vi "Make DriveBase Curves.vi"() -> ()   [LabVIEW 2020]
uses:
  Motor Type.ctl
panel:
  in  "Count":dbl
  in  "Robot Characterization":T1={"Total Mass"=68.0388555, "Wheel Friction"=1.0, "Wheel Diameter"=0.15239999999999998}
  out "Accel vs Distance for T seconds":T2(graph)
  out "Speed vs Distance for T seconds":T3(graph)
  in  "Ratio":dbl
  in  "Masses":T4(array[cluster])
  out "Accel vs Distance for T seconds":T2(graph)
  in  "Loop Time":dbl[unit]=1.0
  out "Speed vs Distance for T seconds":T3(graph)
  in  "Ratios":dbl[](array[numeric])
  in  "Motor Type":T5=enum."Neo"
  # "Robot Sprint for this many seconds"
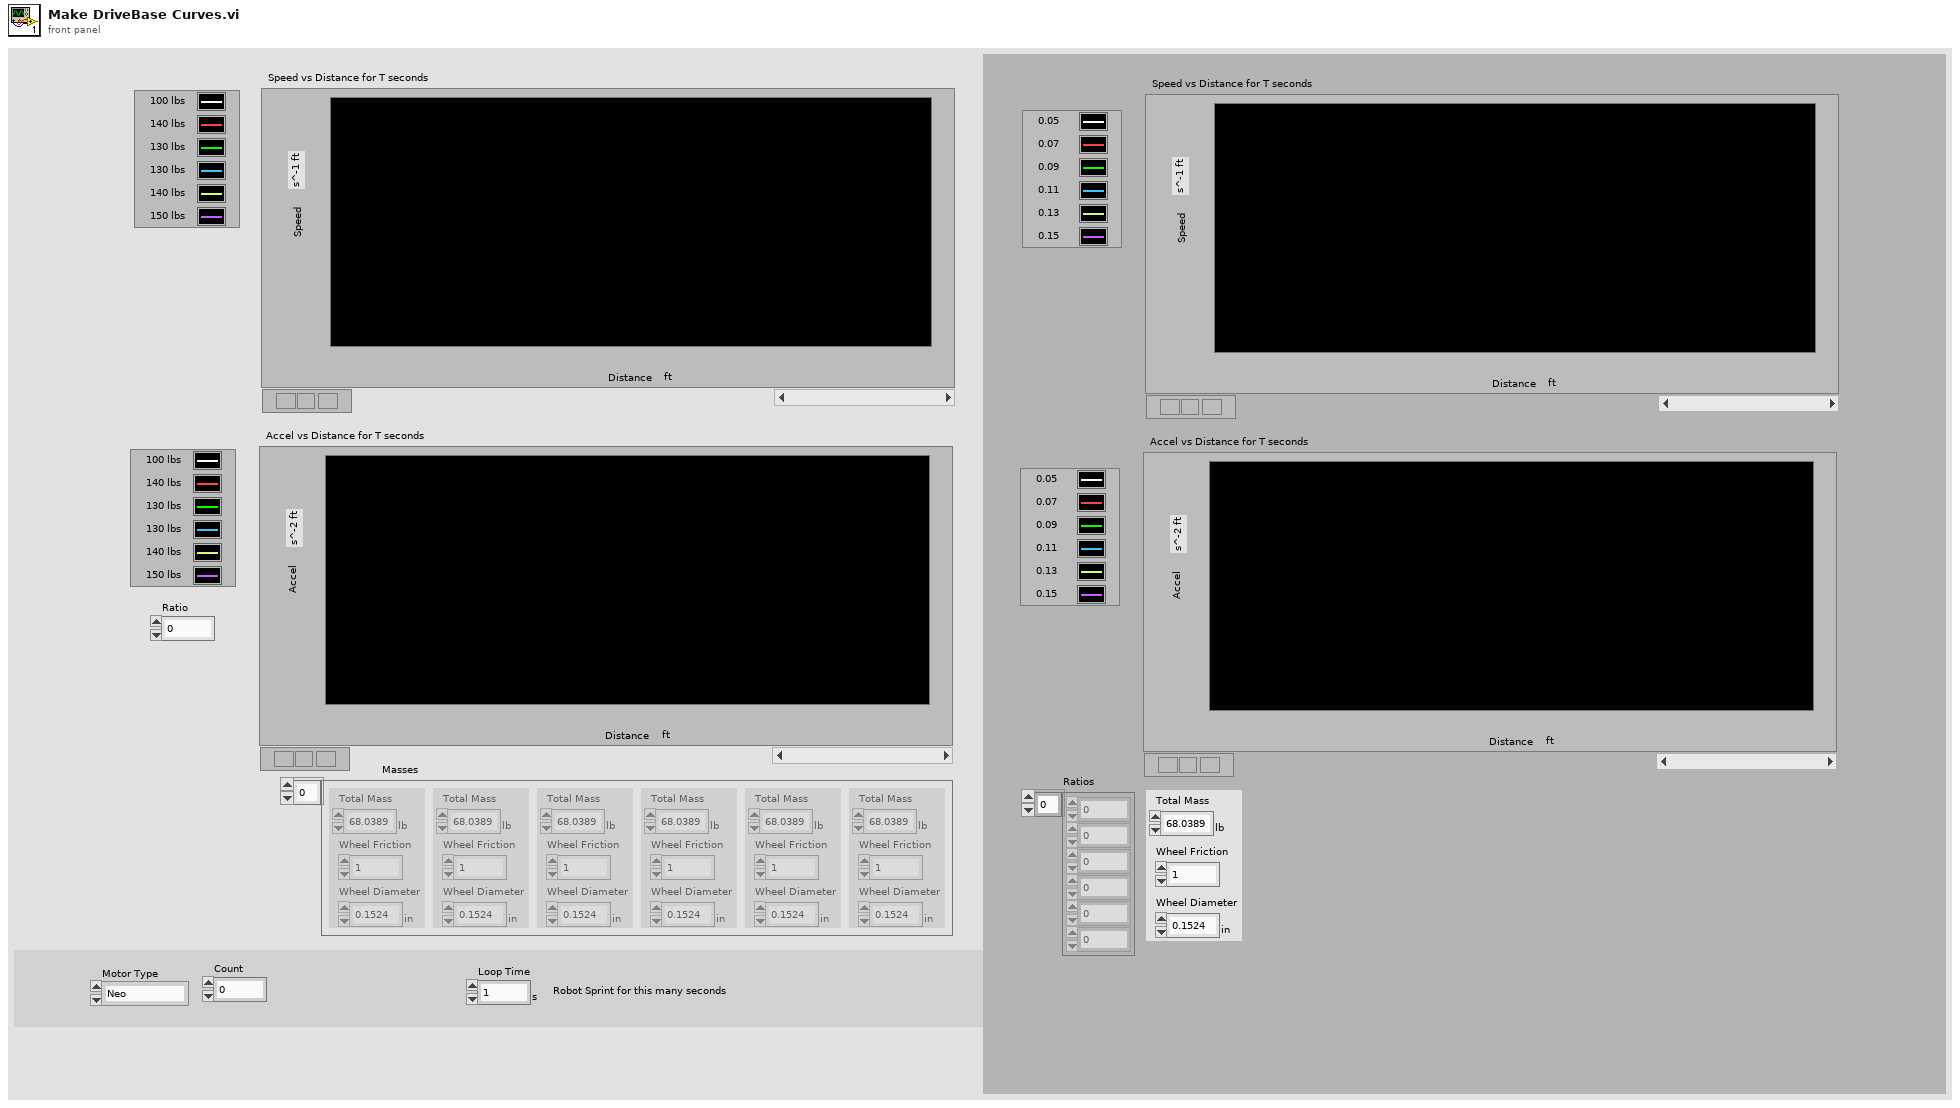
[diagram p1: front panel]
types:
  T1 = cluster{"Total Mass":dbl[unit], "Wheel Friction":dbl, "Wheel Diameter":dbl[unit]}
  T2 = cluster{cluster{"Distance":dbl[unit], "Accel":dbl[unit]}[]}[]
  T3 = cluster{cluster{"Distance":dbl[unit], "Velocity":dbl[unit]}[]}[]
  T4 = cluster{"Total Mass":dbl[unit], "Wheel Friction":dbl, "Wheel Diameter":dbl[unit]}[]
  T5 = typedef "Motor Type.ctl" = enum16{"Custom", "775 pro", "CIM", "miniCIM", "Neo", "Neo 550", "Falcon 500"}
  T6 = cluster{dbl[unit], cluster{"Distance":dbl[unit], "Accel":dbl[unit], "Velocity":dbl[unit]}}[]
  T7 = cluster{"Total Mass":dbl[unit], "Array":cluster{dbl[unit], cluster{"Distance":dbl[unit], "Accel":dbl[unit], "Velocity":dbl[unit]}}[]}
  T8 = cluster{"Numeric":dbl, "Array":cluster{dbl[unit], cluster{"Distance":dbl[unit], "Accel":dbl[unit], "Velocity":dbl[unit]}}[]}
  T9 = cluster{"Distance":dbl[unit], "Accel":dbl[unit], "Velocity":dbl[unit]}
  T10 = cluster{"Distance":dbl[unit], "Velocity":dbl[unit]}
  T11 = cluster{cluster{"Distance":dbl[unit], "Accel":dbl[unit]}[]}
  T12 = cluster{cluster{"Distance":dbl[unit], "Velocity":dbl[unit]}[]}
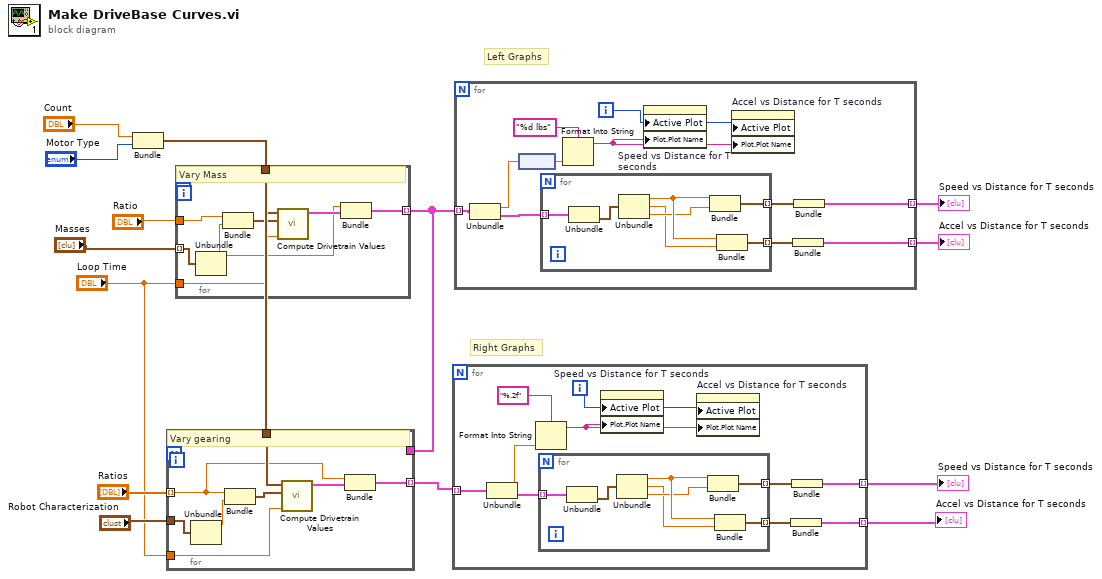
[diagram p0: block diagram]
diagram:
  # "Right Graphs"
  # "Left Graphs"
  n1 = Bundle("Count"="Count", "Motor Type"="Motor Type") -> (w1:cluster{"Count":dbl, "Motor Type":T5})  [unwired: 1 in]
  n2 = for {
    tunnel: w1 -> [w22]
    tunnel: "Loop Time" -> [w21]
    tunnel: "Ratio" -> [w16]
    tunnel: [w19] -> w4 mode=indexing
    tunnel: "Masses" -> [w18] mode=indexing
    # "Vary Mass"
    n3 = Unbundle(w18) -> ("Total Mass"=w15:dbl[unit])  [unwired: 2 out]
    n4 = Bundle("Ratio"=w16, "Total Mass"=w15) -> (w17:cluster{"Ratio":dbl, "Total Mass":dbl[unit]})  [unwired: 1 in]
    n5 = call "Compute Drivetrain Values.vi"("Motor count & type"=w22, "ratio & mass"=w17, "Loop Time"=w21) -> ("Array"=w20:T6)  [unwired: 7 in]
    n6 = Bundle("Total Mass"=w15, "Array"=w20) -> (w19:T7)  [unwired: 1 in]
  }
  n7 = for {
    tunnel: w1 -> [w30]
    tunnel: "Loop Time" -> [w29]
    tunnel: "Ratios" -> [w25] mode=indexing
    tunnel: [w27] -> w7 mode=indexing
    tunnel: "Robot Characterization" -> [w26]
    tunnel: w4 -> [_]
    # "Vary gearing"
    n8 = Unbundle(w26) -> ("Total Mass"=w24:dbl[unit])  [unwired: 2 out]
    n9 = Bundle("Numeric"=w25, "Total Mass"=w24) -> (w23:cluster{"Numeric":dbl, "Total Mass":dbl[unit]})  [unwired: 1 in]
    n10 = call "Compute Drivetrain Values.vi"("Motor count & type"=w30, "ratio & mass"=w23, "Loop Time"=w29) -> ("Array"=w28:T6)  [unwired: 7 in]
    n11 = Bundle("Numeric"=w25, "Array"=w28) -> (w27:T8)  [unwired: 1 in]
  }
  n12 = for {
    tunnel: w7 -> [w40] mode=indexing
    tunnel: [w37] -> w6 mode=indexing
    tunnel: [w35] -> w5 mode=indexing
    i -> [w34]
    n13 = Unbundle(w40) -> ("Numeric"=w32:dbl, "Array"=w39:T6)
    n14 = Format Into String(format string="%.2f", w32) -> (resulting string=w33:string)  [unwired: 2 in, 1 out]
    n15 = for {
      tunnel: w39 -> [w47] mode=indexing
      tunnel: [w45] -> w38 mode=indexing
      tunnel: [w44] -> w36 mode=indexing
      n16 = Unbundle(w47) -> (w46:T9)  [unwired: 1 out]
      n17 = Unbundle(w46) -> ("Distance"=w43:dbl[unit], "Accel"=w41:dbl[unit], "Velocity"=w42:dbl[unit])
      n18 = Bundle("Distance"=w43, "Velocity"=w42) -> (w45:T10)  [unwired: 1 in]
      n19 = Bundle("Distance"=w43, "Accel"=w41) -> (w44:cluster{"Distance":dbl[unit], "Accel":dbl[unit]})  [unwired: 1 in]
    }
    n20 = property on="Speed vs Distance for T seconds" class="XYGraph (strict)"("Active Plot"=w34, "Plot.Plot Name"=w33) -> ()  [unwired: 2 in, 2 out]
    n21 = property on="Accel vs Distance for T seconds" class="XYGraph (strict)"("Active Plot"=w34, "Plot.Plot Name"=w33) -> ()  [unwired: 2 in, 2 out]
    n22 = Bundle(w36) -> (w35:T11)  [unwired: 1 in]
    n23 = Bundle(w38) -> (w37:T12)  [unwired: 1 in]
  }
  "Speed vs Distance for T seconds" <- w6
  "Accel vs Distance for T seconds" <- w5
  n24 = for {
    tunnel: w4 -> [w58] mode=indexing
    tunnel: [w55] -> w14 mode=indexing
    tunnel: [w53] -> w13 mode=indexing
    i -> [w49]
    n25 = Unbundle(w58) -> ("Total Mass"=w52:dbl[unit], "Array"=w57:T6)
    n26 = node(w52) -> (w51:dbl)
    n27 = for {
      tunnel: w57 -> [w65] mode=indexing
      tunnel: [w63] -> w56 mode=indexing
      tunnel: [w62] -> w54 mode=indexing
      n28 = Unbundle(w65) -> (w64:T9)  [unwired: 1 out]
      n29 = Unbundle(w64) -> ("Distance"=w61:dbl[unit], "Accel"=w59:dbl[unit], "Velocity"=w60:dbl[unit])
      n30 = Bundle("Distance"=w61, "Velocity"=w60) -> (w63:T10)  [unwired: 1 in]
      n31 = Bundle("Distance"=w61, "Accel"=w59) -> (w62:cluster{"Distance":dbl[unit], "Accel":dbl[unit]})  [unwired: 1 in]
    }
    n32 = Format Into String(format string="%d lbs", w51) -> (resulting string=w48:string)  [unwired: 2 in, 1 out]
    n33 = property on="Speed vs Distance for T seconds" class="XYGraph (strict)"("Active Plot"=w49, "Plot.Plot Name"=w48) -> ()  [unwired: 2 in, 2 out]
    n34 = property on="Accel vs Distance for T seconds" class="XYGraph (strict)"("Active Plot"=w49, "Plot.Plot Name"=w48) -> ()  [unwired: 2 in, 2 out]
    n35 = Bundle(w54) -> (w53:T11)  [unwired: 1 in]
    n36 = Bundle(w56) -> (w55:T12)  [unwired: 1 in]
  }
  "Speed vs Distance for T seconds" <- w14
  "Accel vs Distance for T seconds" <- w13
